vi "Run.vi"(8 "Error In":errorcluster, 10 "Frame Count":u64, 11 "Shooting Stars In":refnum<class "Shooting Stars.lvclass">) -> (0 "Error Out":errorcluster, 2 "Display Elements":refnum<class "Display Element.lvclass">[](array[class]), 3 "Shooting Stars Out":refnum<class "Shooting Stars.lvclass">)   [LabVIEW 2021, in "Shooting Stars.lvclass"]
uses:
  Shooting Stars.lvclass
  Display Element/Display Element.lvclass
  Pixel/Pixel.lvclass
  C:/Git/MEMOSFET/myRIO-Neopixel/Source/RT/Display Element/Display Element.lvclass
  <vilib>/numeric/Random Number (Range) I64.vi
  <vilib>/numeric/sub_Random U32.vi
  Shooting Stars.lvclass/Shooting Stars.ctl
  C:/Git/MEMOSFET/myRIO-Neopixel/Source/RT/Pixel/Pixel.lvclass
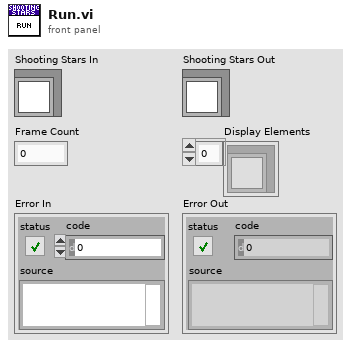
[diagram p1: front panel]
types:
  T1 = typedef "Display Utilities.lvlib/2D Coordinates.ctl" = cluster{"X":i32, "Y":i32}
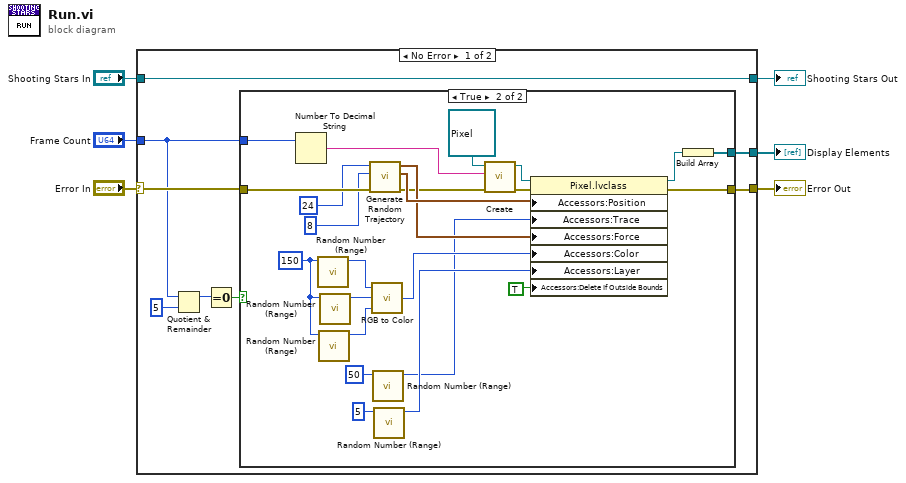
[diagram p0: block diagram]
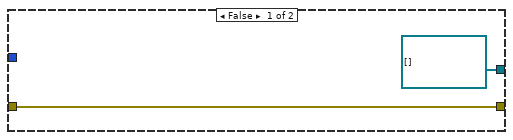
[diagram p2: hidden frame]
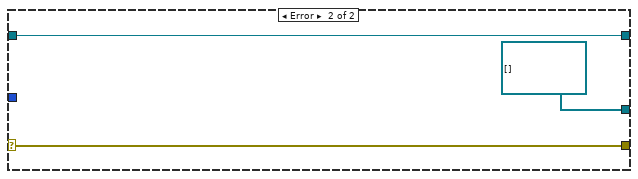
[diagram p3: hidden frame]
diagram:
  n1 = case shown="No Error" "Error In" {
    selector: "Error In" -> [w10 w42]
    tunnel: "Shooting Stars In" -> [w14 w43]
    tunnel: [w9 w42] -> w6
    tunnel: [w14 w43] -> w4
    tunnel: [w7 refnum<class "Display Element.lvclass">[] [] ("Display Elements")] -> w5
    tunnel: "Frame Count" -> [w8 _]
    frame No Error {
      n2 = Quotient & Remainder(x=w8, y=u64 5) -> (x-y*floor(x/y)=w12:u64)  [unwired: 1 out]
      n3 = Equal To 0?(x=w12) -> (x = 0?=w11:bool)
      n4 = case shown="True" w11 {
        tunnel: w10 -> [w16 w29]
        tunnel: w8 -> [_ w40]
        tunnel: [w16 w32] -> w9
        tunnel: [refnum<class "Pixel.lvclass">[] [] w30] -> w7
        frame False {
        }
        frame True {
          w19 = i64 150 ("upper bound (100)")
          n5 = Number To Decimal String(number=w40) -> (decimal integer string=w35:string)  [unwired: 1 in]
          n6 = call-poly <vilib>:"Random Number (Range).vi"("upper bound (100)"=w19) -> ("number"=w22:i64)  [unwired: 10 in]
          n7 = call-poly <vilib>:"Random Number (Range).vi"("upper bound (100)"=w19) -> ("number"=w20:i64)  [unwired: 10 in]
          n8 = call-poly <vilib>:"Random Number (Range).vi"("upper bound (100)"=w19) -> ("number"=w21:i64)  [unwired: 10 in]
          n9 = call "Generate Random Trajectory.vi"("Error In"=w29, "Height"=u64 8, "Width"=u64 24) -> ("Error Out"=w28:errorcluster, "Position"=w39:T1, "Force"=w38:T1)  [unwired: 6 in]
          n10 = call <vilib>:"RGB to Color.vi"("B"=w20, "G"=w21, "R"=w22) -> ("Color"=w23:u32)
          n11 = call-poly <vilib>:"Random Number (Range).vi"("upper bound (100)"=i64 50) -> ("number"=w17:i64)  [unwired: 10 in]
          n12 = call-poly <vilib>:"Random Number (Range).vi"("upper bound (100)"=i64 5) -> ("number"=w25:i64)  [unwired: 10 in]
          n13 = call-dynamic "Create.vi"("Error In"=w28, "Tag"=w35, "Pixel In"=refnum<class "Pixel.lvclass"> refnum ("Pixel.lvclass")) -> ("Error Out"=w33:errorcluster, "Pixel Out"=w34:refnum<class "Pixel.lvclass">)  [unwired: 7 in]
          n14 = property class="Pixel.lvclass"(reference=w34, error in=w33, "Accessors:Position"=w39, "Accessors:Trace"=w17, "Accessors:Force"=w38, "Accessors:Color"=w23, "Accessors:Layer"=w25, "Accessors:Delete If Outside Bounds"=TRUE ("Delete If Outside Bounds")) -> (reference out=w31:refnum<class "Pixel.lvclass">, error out=w32:errorcluster)
          n15 = Build Array(w31) -> (w30:refnum<class "Pixel.lvclass">[])
        }
      }
    }
    frame Error {
    }
  }
  "Shooting Stars Out" <- w4
  "Error Out" <- w6
  "Display Elements" <- w5
